vi "Window-Pockels cal file load.vi"() -> ()   [LabVIEW 2017]
uses:
  Configuration code/Calibration/Globals/gl_Calibration globals.vi
  Global Variables/General Globals.vi
panel:
  in  "Close":bool
  in  "Browse button":bool
  out "Loaded file":string caption="Active Pockels calibration file"
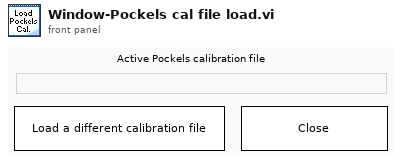
[diagram p1: front panel]
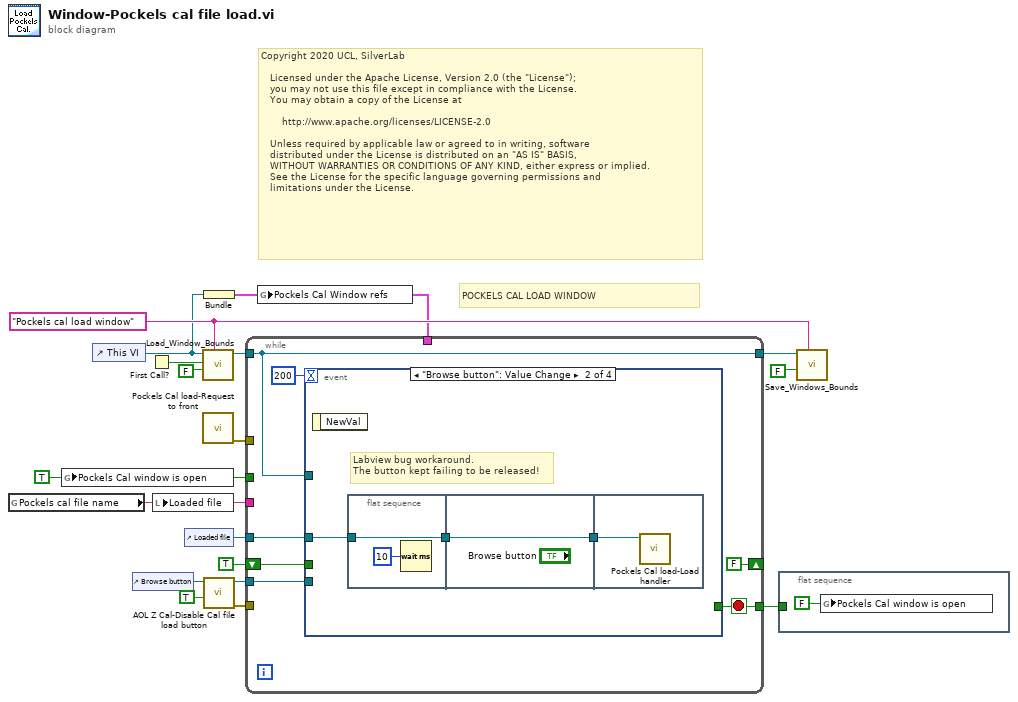
[diagram p0: block diagram]
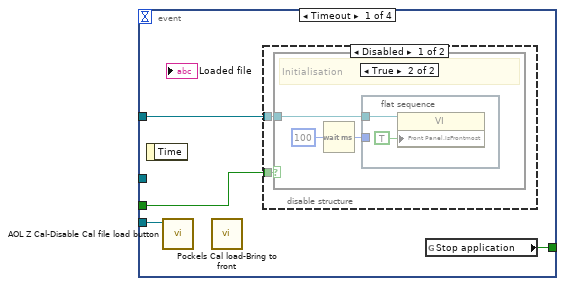
[diagram p2: hidden frame]
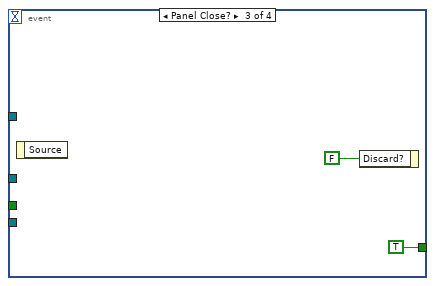
[diagram p5: hidden frame]
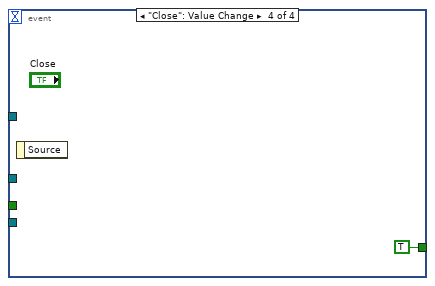
[diagram p6: hidden frame]
diagram:
  w12 = TRUE ("Motor Z calibr window is open")
  w17 = "Pockels cal load window" ("Window Name (i.e. Key)")
  # "Copyright 2020 UCL, SilverLab\n \n   Licensed under the Apache License, Version 2.0 (the \"License\");\n   you may not use this file except in compliance with the License.\n   You may obtain a copy of the License at\n \n       http://www.apache.org/licenses/LICENSE-2.0\n \n   Unless required by applicable law or agreed to in writing, software\n   distributed under the License is distributed on an \"AS IS\" BASIS,\n   WITHOUT WARRANTIES OR CONDITIONS OF ANY KIND, either express or implied.\n   See the License for the specific language governing permissions and\n   limitations under the License."
  # "POCKELS CAL LOAD WINDOW"
  n1 = global read "gl_Calibration globals.vi" "Pockels cal file name"() -> (w1:string)
  n2 = global write "gl_Calibration globals.vi" "Pockels Cal window is open"(w12) -> ()
  n3 = control-ref of="This VI"() -> (w11:refnum<vi>)
  n4 = control-ref of="Browse button"() -> (w5:refnum<vi>)
  n5 = First Call?() -> (First Call?: T/F=w14:bool)
  n6 = local write "Loaded file"(w1) -> ()
  n7 = control-ref of="Loaded file"() -> (w8:refnum<vi>)
  n8 = call "Load_Window_Bounds.vi"("Window Name (i.e. Key)"=w17, "Disable"=FALSE, "First Call"=w14, "Window VI's Ref"=w11) -> ("reference out"=w16:refnum<vi>)  [unwired: 4 in, 3 out]
  n9 = call "Pockels Cal load-Request to front.vi"() -> ("error out"=w9:errorcluster)  [unwired: 11 in]
  n10 = Bundle("This VI"=w11) -> (w10:cluster{"This VI":refnum<vi>})  [unwired: 1 in]
  n11 = call "AOL Z Cal-Disable Cal file load button.vi"("Init"=TRUE, "Browse button ref"=w5) -> ("error out"=w3:errorcluster, "Browse button ref"=w2:refnum<vi>)  [unwired: 8 in]
  n12 = while {
    tunnel: [w24] -> w18
    tunnel: w16 -> [w22]
    tunnel: [w22] -> w15
    tunnel: w12 -> [_]
    tunnel: w10 -> [_]
    tunnel: w9 -> [_]
    tunnel: w1 -> [_]
    tunnel: w8 -> [w23]
    shift-right: [FALSE] -> _
    shift-left: TRUE -> [w21]
    tunnel: w3 -> [_]
    tunnel: w2 -> [w19]
    stop <- w24 stop-if-true
    n13 = event shown="[1] \"Browse button\": Value Change" {
      selector: _ -> [_ _ _ _]
      dyn-events: _ -> [_ _ _ _]
      timeout: 200 -> [_ _ _ _]
      tunnel: [w29 _ TRUE TRUE ("Stop application")] -> w24
      tunnel: w23 -> [_ w39 _ _]
      tunnel: w22 -> [w28 _ _ _]
      tunnel: w21 -> [w27 _ _ _]
      tunnel: w19 -> [w26 _ _ _]
      event Timeout {
        n14 = event-data() -> ()  [unwired: 1 in, 1 out]
        n15 = call "AOL Z Cal-Disable Cal file load button.vi"("Browse button ref"=w26) -> ()  [unwired: 9 in, 2 out]
        n16 = call "Pockels Cal load-Bring to front.vi"() -> ()  [unwired: 12 in]
        n17 = disable-structure shown="Disabled" {
          disable-tunnel: w28 -> [w31 _]
          disable-tunnel: w27 -> [w30 _]
          frame Disabled {
            n18 = case shown="True" w30 {
              tunnel: w31 -> [_ w34]
              frame False {
              }
              frame True {
                # "Initialisation"
                n19 = Wait (ms)(milliseconds to wait=u32 100) -> (millisecond timer value=w32:u32)
                n20 = flat-sequence {
                  tunnel: w34 -> [w35]
                  tunnel: w32 -> [_]
                  frame #0 {
                    n21 = property on="Property Node" class="VI"(reference=w35, "Front Panel.IsFrontmost"=TRUE ("Front Panel Window:Is Frontmost")) -> ()  [unwired: 1 in, 2 out]
                  }
                }
              }
            }
          }
          frame Enabled {
          }
        }
        n22 = global read "General Globals.vi" "Stop application"() -> (w29:bool)
      }
      event "Browse button": Value Change {
        # "Labview bug workaround.\nThe button kept failing to be released!"
        n23 = event-data() -> ()  [unwired: 1 in, 1 out]
        n24 = flat-sequence {
          tunnel: w39 -> [w41]
          tunnel: [w41] -> w37
          tunnel: [w42] -> w38
          tunnel: w37 -> [w42]
          tunnel: w38 -> [w43]
          frame #0 {
            n25 = Wait (ms)(milliseconds to wait=u32 10) -> ()  [unwired: 1 out]
          }
          frame #1 {
          }
          frame #2 {
            n26 = call "Pockels Cal load-Load handler.vi"("Loaded pockels cal file"=w43) -> ()  [unwired: 11 in]
          }
        }
      }
      event Panel Close? {
        n27 = event-data() -> ()  [unwired: 1 in, 1 out]
        n28 = event-data("Discard?"=FALSE) -> ()  [unwired: 1 in, 1 out]
      }
      event "Close": Value Change {
        n29 = event-data() -> ()  [unwired: 1 in, 1 out]
      }
    }
  }
  n30 = global write "gl_Calibration globals.vi" "Pockels Cal Window refs"(w10) -> ()
  n31 = flat-sequence {
    tunnel: w18 -> [_]
    frame #0 {
      n32 = global write "gl_Calibration globals.vi" "Pockels Cal window is open"(FALSE ("Motor Z calibr window is open")) -> ()
    }
  }
  n33 = call "Save_Windows_Bounds.vi"("Window Name (i.e. Key)"=w17, "Front Panel Window:Open"=FALSE ("Disable"), "Window VI's Ref"=w15) -> ()  [unwired: 8 in, 1 out]
